vi "Message(9600).vi"(7 "Число каналов":i32=12) -> (8 "Channels":cluster{dbl, i32, bool[], "Type":i32}[](array[cluster]), 10 "Message":bool[][](array[boolean]))   [LabVIEW 2013]
panel:
  in  "Amplitude":dbl=0.5
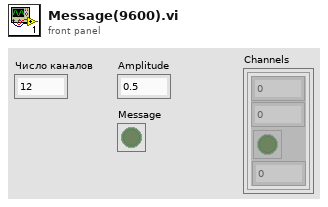
[diagram p1: front panel]
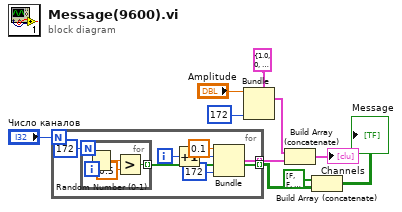
[diagram p0: block diagram]
diagram:
  n1 = for {
    N: "Число каналов" -> [_]
    tunnel: [w15] -> w9 mode=indexing
    tunnel: [w12] -> w6 mode=indexing
    i -> [w14]
    n2 = for {
      N: 172 -> [_]
      tunnel: [w18] -> w12 mode=indexing
      n3 = Random Number (0-1)() -> (number: 0 to 1=w20:dbl)
      n4 = Greater?(x=w20, y=0.5) -> (0:w18:bool)
    }
    n5 = Increment(x=w14) -> (x+1=w13:i32)
    n6 = Bundle(0.1, w13, w12, 172) -> (w15:cluster{dbl, i32, bool[], i32})  [unwired: 1 in]
  }
  n7 = Bundle(cluster=cluster{dbl, i32, bool[], "Type":i32} {1.0, 0, [FALSE, FALSE, FALSE, FALSE, FALSE, FALSE, FALSE, FALSE, FALSE, FALSE, FALSE, FALSE, FALSE, FALSE, FALSE, FALSE, FALSE, FALSE, FALSE, FALSE, FALSE, FALSE, FALSE, FALSE, FALSE, FALSE, FALSE, FALSE, FALSE, FALSE, FALSE, FALSE, FALSE, FALSE, FALSE, FALSE, FALSE, FALSE, FALSE, FALSE, FALSE, FALSE, FALSE, FALSE, FALSE, FALSE, FALSE, FALSE, FALSE, FALSE, FALSE, FALSE, FALSE, FALSE, FALSE, FALSE, FALSE, FALSE, FALSE, FALSE, FALSE, FALSE, FALSE, FALSE, FALSE, FALSE, FALSE, FALSE, FALSE, FALSE, FALSE, FALSE, FALSE, FALSE, FALSE, FALSE, FALSE, FALSE, FALSE, FALSE], "Type"=80} ("Frame(PICH) 2"), "Amplitude", "Type"=172) -> (w8:cluster{dbl, i32, bool[], "Type":i32})  [unwired: 2 in]
  n8 = Build Array (concatenate)(w8, w9) -> (→"Channels":cluster{dbl, i32, bool[], "Type":i32}[])
  n9 = Build Array (concatenate)(bool[] [FALSE, FALSE, FALSE, FALSE, FALSE, FALSE, FALSE, FALSE, FALSE, FALSE, FALSE, FALSE, FALSE, FALSE, FALSE, FALSE, FALSE, FALSE, FALSE, FALSE, FALSE, FALSE, FALSE, FALSE, FALSE, FALSE, FALSE, FALSE, FALSE, FALSE, FALSE, FALSE, FALSE, FALSE, FALSE, FALSE, FALSE, FALSE, FALSE, FALSE, FALSE, FALSE, FALSE, FALSE, FALSE, FALSE, FALSE, FALSE, FALSE, FALSE, FALSE, FALSE, FALSE, FALSE, FALSE, FALSE, FALSE, FALSE, FALSE, FALSE, FALSE, FALSE, FALSE, FALSE, FALSE, FALSE, FALSE, FALSE, FALSE, FALSE, FALSE, FALSE, FALSE, FALSE, FALSE, FALSE, FALSE, FALSE, FALSE, FALSE, FALSE, FALSE, FALSE, FALSE, FALSE, FALSE, FALSE, FALSE, FALSE, FALSE, FALSE, FALSE, FALSE, FALSE, FALSE, FALSE, FALSE, FALSE, FALSE, FALSE, FALSE, FALSE, FALSE, FALSE, FALSE, FALSE, FALSE, FALSE, FALSE, FALSE, FALSE, FALSE, FALSE, FALSE, FALSE, FALSE, FALSE, FALSE, FALSE, FALSE, FALSE, FALSE, FALSE, FALSE, FALSE, FALSE, FALSE, FALSE, FALSE, FALSE, FALSE, FALSE, FALSE, FALSE, FALSE, FALSE, FALSE, FALSE, FALSE, FALSE, FALSE, FALSE, FALSE, FALSE, FALSE, FALSE, FALSE, FALSE, FALSE, FALSE, FALSE, FALSE, FALSE, FALSE, FALSE, FALSE, FALSE, FALSE, FALSE, FALSE, FALSE, FALSE, FALSE, FALSE, FALSE, FALSE, FALSE, FALSE, FALSE, FALSE, FALSE, FALSE] ("Array 2"), w6) -> (→"Message":bool[][])
